vi "Save MPU calib.vi"(7 "Calib data type":T1(ring), 8 "Error In":errorcluster, 10 "Calib data":sgl[](array[numeric])) -> (0 "Error Out":errorcluster)   [LabVIEW 2016]
uses:
  <vilib>/Utility/config.llb/Write Key (Double).vi
  <vilib>/Utility/config.llb/NI_LVConfig.lvlib
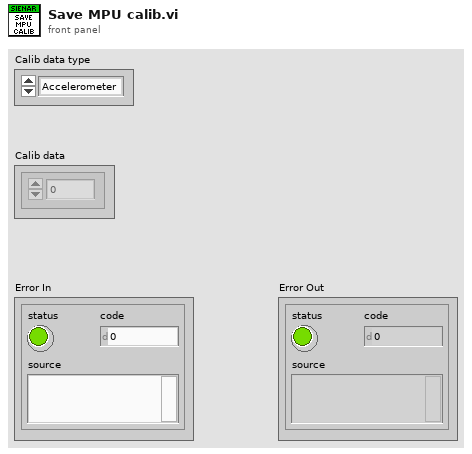
[diagram p1: front panel]
types:
  T1 = enum16{"Accelerometer", "Gyroscope", "Magnetometer"}
  T2 = typedef "NI_LVConfig.lvlib/Config Data RefNum.ctl" = refnum<k1>
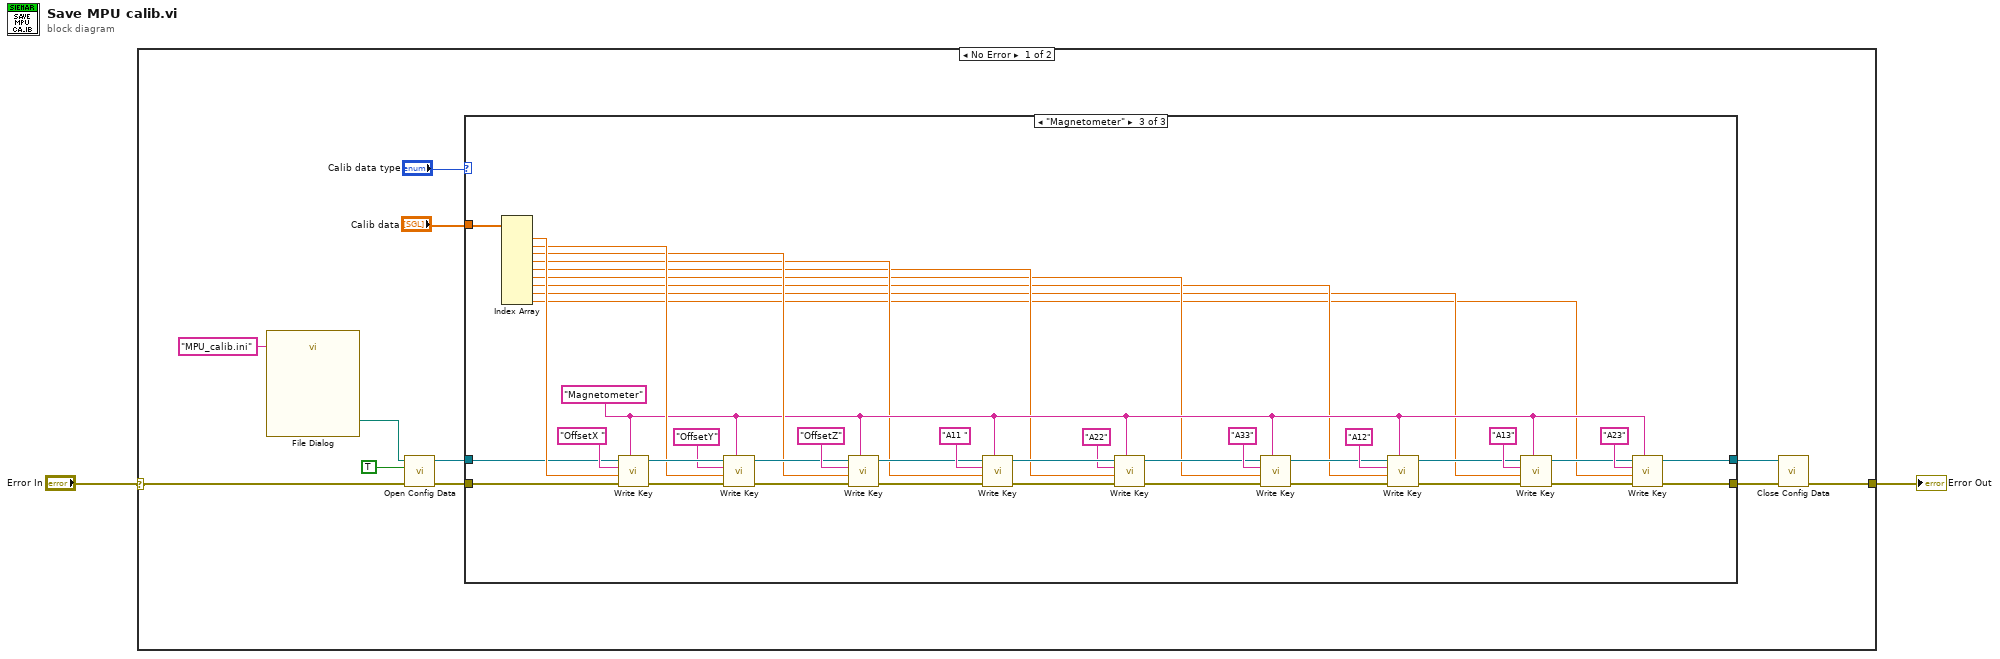
[diagram p0: block diagram]
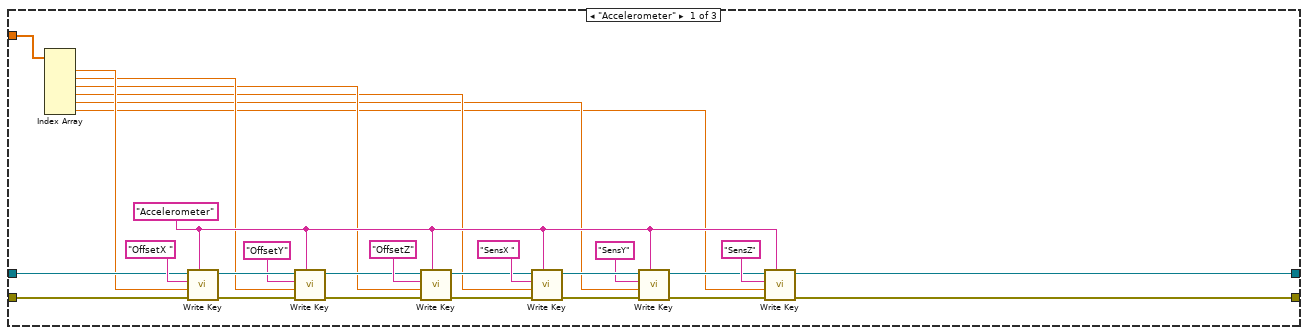
[diagram p2: hidden frame]
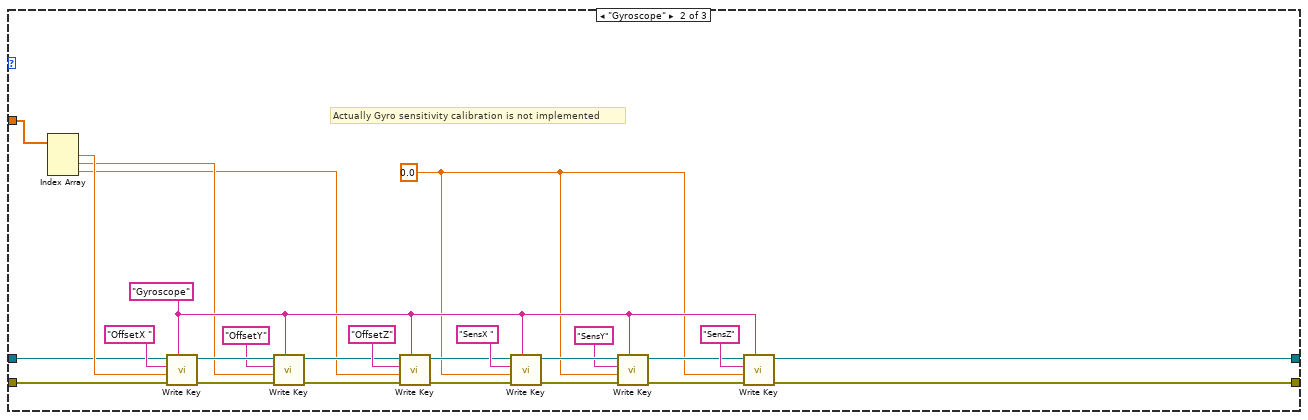
[diagram p3: hidden frame]
diagram:
  n1 = case shown="No Error" "Error In" {
    selector: "Error In" -> [w3 w108]
    tunnel: [w6 w108] -> w2
    frame No Error {
      n2 = call "File Dialog"("default name"="MPU_calib.ini") -> ("selected path"=w5:path)  [unwired: 11 in, 3 out]
      n3 = call <vilib>:"Open Config Data.vi"("error in (no error)"=w3, "create file if necessary (T)"=TRUE, "configuration file path"=w5) -> ("error out"=w10:errorcluster, "refnum"=w9:T2)  [unwired: 6 in, 1 out]
      n4 = case shown="\"Magnetometer\"" "Calib data type" {
        tunnel: "Calib data" -> [w22 w45 w81]
        tunnel: w10 -> [w33 w46 w89]
        tunnel: w9 -> [w34 w47 w90]
        tunnel: [w15 w44 w82] -> w8
        tunnel: [w14 w43 w83] -> w7
        frame "Accelerometer" {
          w21 = "Accelerometer" ("section")
          n5 = Index Array(array=w22) -> (element #1=w32:sgl, element #2=w20:sgl, element #3=w19:sgl, element #4=w18:sgl, element #5=w17:sgl, element #6=w16:sgl)  [unwired: 6 in]
          n6 = call-poly <vilib>:"Write Key.vi"("section"=w21, "error in (no error)"=w33, "value"=w32, "key"="OffsetX ", "refnum"=w34) -> ("error out"=w39:errorcluster, "refnum out"=w40:T2)  [unwired: 4 in, 1 out]
          n7 = call-poly <vilib>:"Write Key.vi"("section"=w21, "error in (no error)"=w39, "value"=w20, "key"="OffsetY", "refnum"=w40) -> ("error out"=w36:errorcluster, "refnum out"=w35:T2)  [unwired: 4 in, 1 out]
          n8 = call-poly <vilib>:"Write Key.vi"("section"=w21, "error in (no error)"=w36, "value"=w19, "key"="OffsetZ", "refnum"=w35) -> ("error out"=w23:errorcluster, "refnum out"=w24:T2)  [unwired: 4 in, 1 out]
          n9 = call-poly <vilib>:"Write Key.vi"("section"=w21, "error in (no error)"=w23, "value"=w18, "key"="SensX ", "refnum"=w24) -> ("error out"=w29:errorcluster, "refnum out"=w30:T2)  [unwired: 4 in, 1 out]
          n10 = call-poly <vilib>:"Write Key.vi"("section"=w21, "error in (no error)"=w29, "value"=w17, "key"="SensY", "refnum"=w30) -> ("error out"=w26:errorcluster, "refnum out"=w25:T2)  [unwired: 4 in, 1 out]
          n11 = call-poly <vilib>:"Write Key.vi"("section"=w21, "error in (no error)"=w26, "value"=w16, "key"="SensZ", "refnum"=w25) -> ("error out"=w14:errorcluster, "refnum out"=w15:T2)  [unwired: 4 in, 1 out]
        }
        frame "Gyroscope" {
          w42 = 0.0
          w50 = "Gyroscope" ("section")
          # "Actually Gyro sensitivity calibration is not implemented"
          n12 = Index Array(array=w45) -> (element #1=w60:sgl, element #2=w49:sgl, element #3=w48:sgl)  [unwired: 3 in]
          n13 = call-poly <vilib>:"Write Key.vi"("section"=w50, "error in (no error)"=w46, "value"=w60, "key"="OffsetX ", "refnum"=w47) -> ("error out"=w65:errorcluster, "refnum out"=w66:T2)  [unwired: 4 in, 1 out]
          n14 = call-poly <vilib>:"Write Key.vi"("section"=w50, "error in (no error)"=w65, "value"=w49, "key"="OffsetY", "refnum"=w66) -> ("error out"=w62:errorcluster, "refnum out"=w61:T2)  [unwired: 4 in, 1 out]
          n15 = call-poly <vilib>:"Write Key.vi"("section"=w50, "error in (no error)"=w62, "value"=w48, "key"="OffsetZ", "refnum"=w61) -> ("error out"=w51:errorcluster, "refnum out"=w52:T2)  [unwired: 4 in, 1 out]
          n16 = call-poly <vilib>:"Write Key.vi"("section"=w50, "error in (no error)"=w51, "value"=w42, "key"="SensX ", "refnum"=w52) -> ("error out"=w57:errorcluster, "refnum out"=w58:T2)  [unwired: 4 in, 1 out]
          n17 = call-poly <vilib>:"Write Key.vi"("section"=w50, "error in (no error)"=w57, "value"=w42, "key"="SensY", "refnum"=w58) -> ("error out"=w54:errorcluster, "refnum out"=w53:T2)  [unwired: 4 in, 1 out]
          n18 = call-poly <vilib>:"Write Key.vi"("section"=w50, "error in (no error)"=w54, "value"=w42, "key"="SensZ", "refnum"=w53) -> ("error out"=w43:errorcluster, "refnum out"=w44:T2)  [unwired: 4 in, 1 out]
        }
        frame "Magnetometer" {
          w76 = "Magnetometer" ("section")
          n19 = Index Array(array=w81) -> (element #1=w91:sgl, element #2=w80:sgl, element #3=w79:sgl, element #4=w73:sgl, element #5=w72:sgl, element #6=w71:sgl, element #7=w70:sgl, element #8=w69:sgl, element #9=w68:sgl)  [unwired: 9 in]
          n20 = call-poly <vilib>:"Write Key.vi"("section"=w76, "error in (no error)"=w89, "value"=w91, "key"="OffsetX ", "refnum"=w90) -> ("error out"=w105:errorcluster, "refnum out"=w106:T2)  [unwired: 4 in, 1 out]
          n21 = call-poly <vilib>:"Write Key.vi"("section"=w76, "error in (no error)"=w105, "value"=w80, "key"="OffsetY", "refnum"=w106) -> ("error out"=w102:errorcluster, "refnum out"=w101:T2)  [unwired: 4 in, 1 out]
          n22 = call-poly <vilib>:"Write Key.vi"("section"=w76, "error in (no error)"=w102, "value"=w79, "key"="OffsetZ", "refnum"=w101) -> ("error out"=w93:errorcluster, "refnum out"=w92:T2)  [unwired: 4 in, 1 out]
          n23 = call-poly <vilib>:"Write Key.vi"("section"=w76, "error in (no error)"=w93, "value"=w73, "key"="A11 ", "refnum"=w92) -> ("error out"=w98:errorcluster, "refnum out"=w99:T2)  [unwired: 4 in, 1 out]
          n24 = call-poly <vilib>:"Write Key.vi"("section"=w76, "error in (no error)"=w98, "value"=w72, "key"="A22", "refnum"=w99) -> ("error out"=w95:errorcluster, "refnum out"=w94:T2)  [unwired: 4 in, 1 out]
          n25 = call-poly <vilib>:"Write Key.vi"("section"=w76, "error in (no error)"=w95, "value"=w71, "key"="A33", "refnum"=w94) -> ("error out"=w77:errorcluster, "refnum out"=w78:T2)  [unwired: 4 in, 1 out]
          n26 = call-poly <vilib>:"Write Key.vi"("section"=w76, "error in (no error)"=w77, "value"=w70, "key"="A12", "refnum"=w78) -> ("error out"=w86:errorcluster, "refnum out"=w85:T2)  [unwired: 4 in, 1 out]
          n27 = call-poly <vilib>:"Write Key.vi"("section"=w76, "error in (no error)"=w86, "value"=w69, "key"="A13", "refnum"=w85) -> ("error out"=w75:errorcluster, "refnum out"=w74:T2)  [unwired: 4 in, 1 out]
          n28 = call-poly <vilib>:"Write Key.vi"("section"=w76, "error in (no error)"=w75, "value"=w68, "key"="A23", "refnum"=w74) -> ("error out"=w83:errorcluster, "refnum out"=w82:T2)  [unwired: 4 in, 1 out]
        }
      }
      n29 = call <vilib>:"Close Config Data.vi"("error in (no error)"=w7, "refnum"=w8) -> ("error out"=w6:errorcluster)  [unwired: 8 in, 1 out]
    }
    frame Error {
    }
  }
  "Error Out" <- w2
